vi "SUB_COM9_ESC.vi"(3 "VISA resource name":refnum<visa-resource-name>) -> (1 "duplicate VISA resource name":refnum<visa-resource-name>)   [LabVIEW 2011]
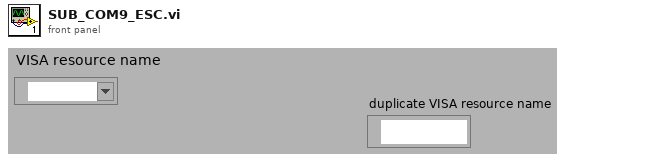
[diagram p1: front panel]
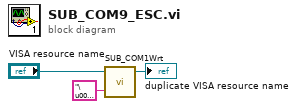
[diagram p0: block diagram]
diagram:
  n1 = call "SUB_COM1Wrt.vi"("VISA resource name"="VISA resource name", "write buffer"="\u001b") -> ("duplicate VISA resource name"=→"duplicate VISA resource name":refnum<visa-resource-name>)  [unwired: 2 out]
